vi "TrapezoidalMotionProfile.vi"(5 "MaxAccel":dbl=75.0, 7 "MaxVelocity":dbl=100.0, 8 "dt":u32=20, 9 "FinalVelocity":dbl, 10 "InitialVelocity":dbl, 11 "Distance":dbl=200.0) -> (0 "dt":u32=20, 3 "Profile":cluster{"Pos":dbl, "Vel":dbl, "Accel":dbl}[](array[cluster]))   [LabVIEW 2016]
panel:
  out "Graph":dbl[][](graph)=[[0.0, 0.015000000000000001, 0.060000000000000005, 0.135, 0.24000000000000002, 0.37500000000000006, 0.54, 0.7350000000000001, 0.9600000000000001, 1.2149999999999999, 1.5000000000000002, 1.815, 2.16, 2.535, 2.9400000000000004, 3.375, 3.8400000000000003, 4.335000000000001, 4.859999999999999, 5.415, 6.000000000000001, 6.614999999999999, 7.26, 7.9350000000000005, 8.64, 9.375, 10.14, 10.935, 11.760000000000002, 12.614999999999998, 13.5, 14.415000000000001, 15.360000000000001, 16.335, 17.340000000000003, 18.375000000000004, 19.439999999999998, 20.535, 21.66, 22.815, 24.000000000000004, 25.215000000000003, 26.459999999999997, 27.734999999999996, 29.04, 30.375000000000004, 31.740000000000002, 33.135000000000005, 34.56, 36.015, 37.5, 39.015, 40.56, 42.135000000000005, 43.74, 45.37500000000001, 47.040000000000006, 48.735000000000014, 50.459999999999994, 52.214999999999996, 54.0, 55.815, 57.660000000000004, 59.535000000000004, 61.440000000000005, 63.37500000000001, 65.34, 67.33333333333334, 69.33333333333334, 71.33333333333334, 73.33333333333334, 75.33333333333333, 77.33333333333333, 79.33333333333333, 81.33333333333333, 83.33333333333333, 85.33333333333333, 87.33333333333334, 89.33333333333334, 91.33333333333334, 93.33333333333334, 95.33333333333334, 97.33333333333334, 99.33333333333334, 101.33333333333333, 103.33333333333333, 105.33333333333333, 107.33333333333333, 109.33333333333333, 111.33333333333334, 113.33333333333334, 115.33333333333334, 117.33333333333334, 119.33333333333334, 121.33333333333334, 123.33333333333334, 125.33333333333331, 127.33333333333333, 129.33333333333331, 131.33333333333331, 133.33333333333331, 135.31833333333338, 137.27333333333337, 139.19833333333338, 141.09333333333336, 142.95833333333337, 144.79333333333338, 146.59833333333336, 148.37333333333336, 150.11833333333337, 151.83333333333337, 153.51833333333337, 155.17333333333337, 156.79833333333337, 158.39333333333337, 159.95833333333337, 161.49333333333334, 162.99833333333333, 164.47333333333336, 165.91833333333335, 167.33333333333334, 168.71833333333336, 170.07333333333335, 171.39833333333334, 172.69333333333336, 173.95833333333334, 175.19333333333336, 176.39833333333337, 177.57333333333335, 178.71833333333336, 179.83333333333334, 180.91833333333335, 181.97333333333336, 182.99833333333336, 183.99333333333337, 184.95833333333334, 185.89333333333335, 186.79833333333335, 187.67333333333335, 188.51833333333335, 189.33333333333334, 190.11833333333334, 190.87333333333333, 191.59833333333333, 192.29333333333335, 192.95833333333334, 193.59333333333333, 194.19833333333335, 194.77333333333334, 195.31833333333333, 195.83333333333334, 196.31833333333333, 196.77333333333334, 197.19833333333335, 197.59333333333333, 197.95833333333334, 198.29333333333335, 198.59833333333333, 198.87333333333333, 199.11833333333334, 199.33333333333334, 199.51833333333335, 199.67333333333335, 199.79833333333335, 199.89333333333335, 199.95833333333334, 199.99333333333334, 199.99833333333333], [0.0, 1.5, 3.0, 4.5, 6.0, 7.5, 9.0, 10.500000000000002, 12.0, 13.5, 15.0, 16.5, 18.0, 19.5, 21.000000000000004, 22.5, 24.0, 25.500000000000004, 27.0, 28.5, 30.0, 31.5, 33.0, 34.5, 36.0, 37.5, 39.0, 40.5, 42.00000000000001, 43.5, 45.0, 46.5, 48.0, 49.5, 51.00000000000001, 52.50000000000001, 54.0, 55.5, 57.0, 58.5, 60.0, 61.50000000000001, 63.0, 64.5, 66.0, 67.5, 69.0, 70.5, 72.0, 73.5, 75.0, 76.5, 78.0, 79.5, 81.0, 82.5, 84.00000000000001, 85.50000000000001, 87.0, 88.5, 90.0, 91.5, 93.0, 94.5, 96.0, 97.5, 99.0, 100.0, 100.0, 100.0, 100.0, 100.0, 100.0, 100.0, 100.0, 100.0, 100.0, 100.0, 100.0, 100.0, 100.0, 100.0, 100.0, 100.0, 100.0, 100.0, 100.0, 100.0, 100.0, 100.0, 100.0, 100.0, 100.0, 100.0, 100.0, 100.0, 100.0, 100.0, 100.0, 100.0, 100.0, 98.5, 97.0, 95.5, 94.0, 92.5, 91.0, 89.49999999999999, 87.99999999999999, 86.49999999999999, 84.99999999999999, 83.49999999999999, 81.99999999999999, 80.49999999999999, 78.99999999999999, 77.49999999999997, 76.00000000000001, 74.50000000000001, 73.00000000000001, 71.5, 70.0, 68.5, 67.0, 65.5, 64.0, 62.5, 61.0, 59.5, 57.99999999999999, 56.49999999999999, 54.99999999999999, 53.49999999999999, 51.99999999999999, 50.499999999999986, 48.999999999999986, 47.499999999999986, 45.999999999999986, 44.499999999999986, 42.999999999999986, 41.49999999999998, 39.99999999999998, 38.500000000000014, 37.000000000000014, 35.500000000000014, 34.000000000000014, 32.5, 31.0, 29.5, 28.0, 26.5, 25.0, 23.5, 22.0, 20.5, 19.0, 17.5, 15.999999999999986, 14.499999999999986, 12.999999999999986, 11.499999999999986, 9.999999999999986, 8.499999999999986, 6.999999999999986, 5.499999999999986, 3.999999999999986, 2.499999999999986, 0.9999999999999716, -0.4999999999999858]]
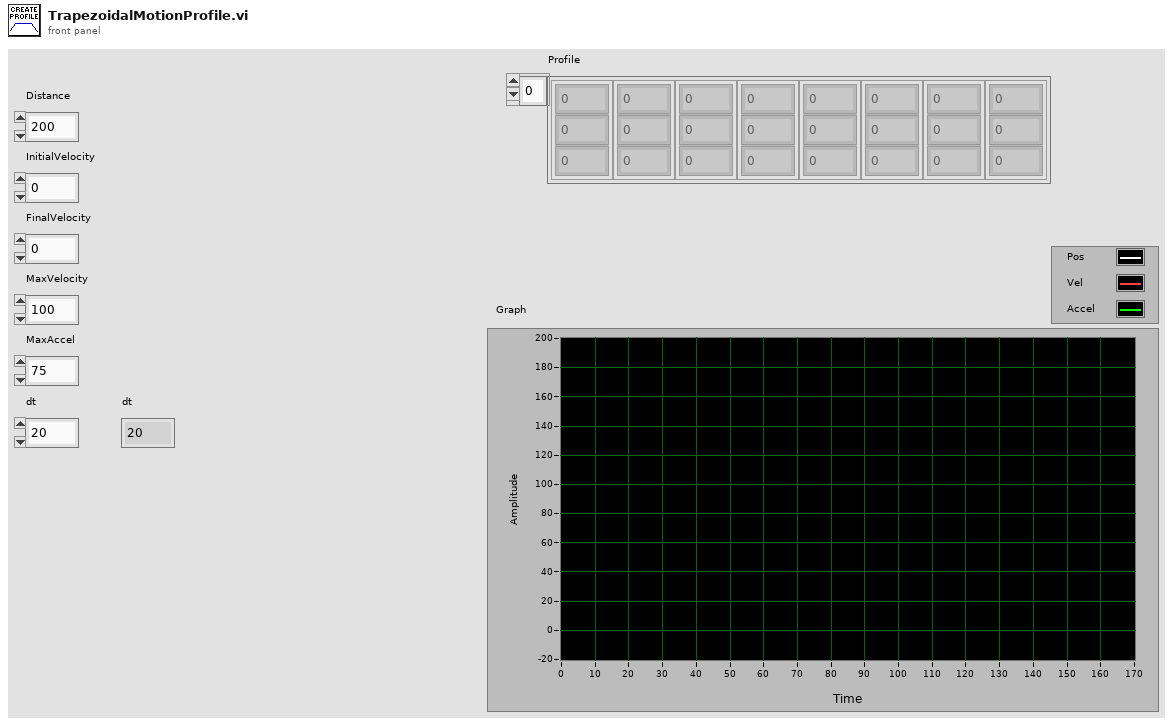
[diagram p1: front panel]
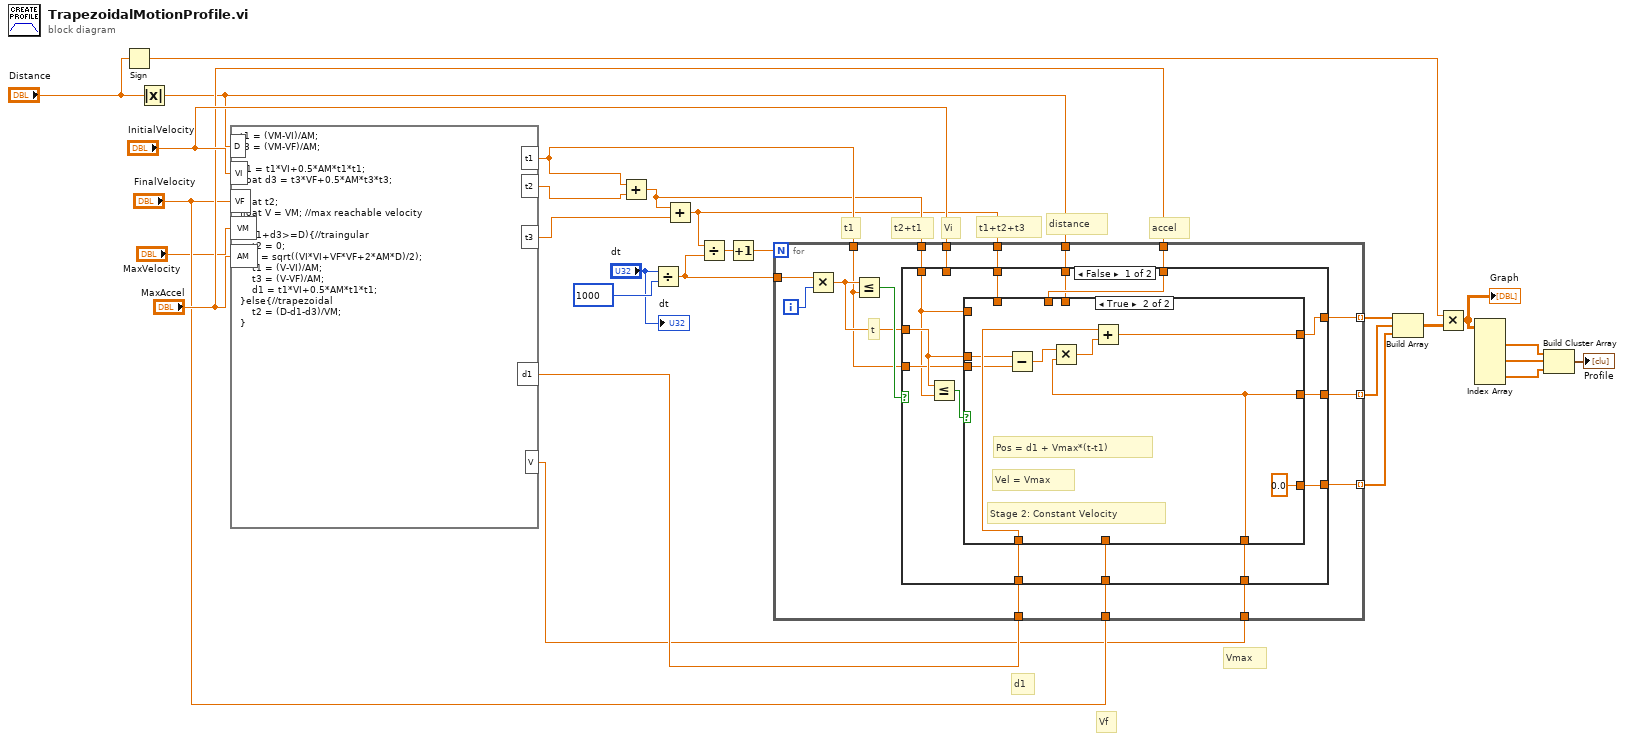
[diagram p0: block diagram]
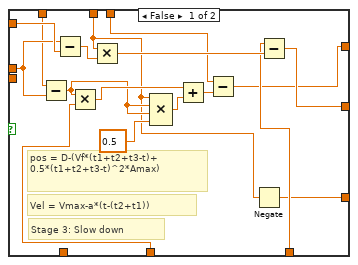
[diagram p2: hidden frame]
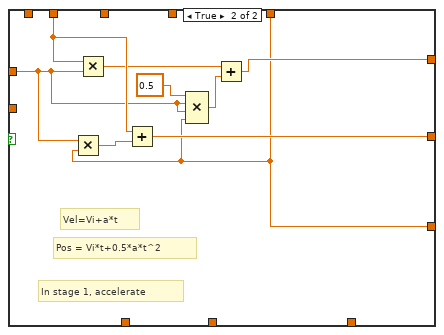
[diagram p3: hidden frame]
diagram:
  # "distance"
  # "Vf"
  # "t1+t2+t3"
  # "d1"
  # "Vmax"
  # "t1"
  # "t2+t1"
  # "Vi"
  # "accel"
  n1 = Sign(1:"Distance") -> (0:w6:dbl)
  n2 = Absolute Value(x="Distance") -> (abs(x)=w9:dbl)
  n3 = formula code="t1 = (VM-VI)/AM;\nt3 = (VM-VF)/AM;\n\nd1 = t1*VI+0.5*AM*t1*t1;\nfloat d3 = t3*VF+0.5*AM*t3*t3;\n\nfloat t2;\nfloat V = VM; //max reachable velocity\n\nif(d1+d3>=D){//traingular\n    t2 = 0;\n    V = sqrt((VI*VI+VF*VF+2*AM*D)/2);\n    t1 = (V-VI)/AM;\n    t3 = (V-VF)/AM;\n    d1 = t1*VI+0.5*AM*t1*t1;\n}else{//trapezoidal\n    t2 = (D-d1-d3)/VM;\n}"("VI"="InitialVelocity", "VF"="FinalVelocity", "D"=w9, "VM"="MaxVelocity", "AM"="MaxAccel") -> ("t1"=w22:dbl, "t3"=w27:dbl, "d1"=w18:dbl, "t2"=w28:dbl, "V"=w11:dbl)
  n4 = Add(x=w22, y=w28) -> (x+y=w19:dbl)
  n5 = Divide(x="dt", y=u32 1000) -> (x/y=w23:dbl)
  n6 = Add(x=w19, y=w27) -> (x+y=w15:dbl)
  n7 = Divide(x=w15, y=w23) -> (x/y=w25:dbl)
  n8 = Increment(x=w25) -> (x+1=w24:dbl)
  n9 = for {
    N: w24 -> [_]
    tunnel: w23 -> [w43]
    tunnel: w22 -> [w33]
    tunnel: "InitialVelocity" -> [w41]
    tunnel: "MaxAccel" -> [w40]
    tunnel: [w39] -> w16 mode=indexing
    tunnel: [w38] -> w17 mode=indexing
    tunnel: w19 -> [w37]
    tunnel: w11 -> [w35]
    tunnel: w18 -> [w34]
    tunnel: w15 -> [w32]
    tunnel: "FinalVelocity" -> [w31]
    tunnel: w9 -> [w30]
    tunnel: [w29] -> w10 mode=indexing
    i -> [w44]
    # "t"
    n10 = Multiply(x=w43, y=w44) -> (x*y=w36:dbl)
    n11 = Less Or Equal?(x=w36, y=w33) -> (x <= y?=w42:bool)
    n12 = case shown="False" w42 {
      tunnel: w41 -> [_ w89]
      tunnel: w40 -> [w49 w83]
      tunnel: w36 -> [w53 w86]
      tunnel: [w56 w90] -> w39
      tunnel: [w51 w84] -> w38
      tunnel: w37 -> [w50 _]
      tunnel: w35 -> [w55 _]
      tunnel: w34 -> [w54 _]
      tunnel: w33 -> [w52 _]
      tunnel: w32 -> [w48 _]
      tunnel: w31 -> [w47 _]
      tunnel: w30 -> [w46 _]
      tunnel: [w45 w83] -> w29
      frame False {
        n13 = Less Or Equal?(x=w53, y=w50) -> (x <= y?=w57:bool)
        n14 = case shown="True" w57 {
          tunnel: [w70 w79] -> w56
          tunnel: w55 -> [w71 w79]
          tunnel: w54 -> [_ w82]
          tunnel: w53 -> [w69 w81]
          tunnel: w52 -> [_ w80]
          tunnel: [w60 w76] -> w51
          tunnel: w50 -> [w74 _]
          tunnel: w49 -> [w58 _]
          tunnel: w48 -> [w68 _]
          tunnel: w47 -> [w67 _]
          tunnel: w46 -> [w61 _]
          tunnel: [w59 0.0] -> w45
          frame False {
            # "pos = D-(Vf*(t1+t2+t3-t)+\n0.5*(t1+t2+t3-t)^2*Amax)"
            # "Vel = Vmax-a*(t-(t2+t1))"
            # "Stage 3: Slow down"
            n15 = Subtract(x=w68, y=w69) -> (x-y=w64:dbl)
            n16 = Subtract(x=w69, y=w74) -> (x-y=w73:dbl)
            n17 = Multiply(x=w64, y=w67) -> (x*y=w66:dbl)
            n18 = Multiply(x=w58, y=w73) -> (x*y=w72:dbl)
            n19 = Compound Arithmetic op=MULTIPLY(w58, w64, w64, 0.5 ("value")) -> (w63:dbl)
            n20 = Add(x=w66, y=w63) -> (x+y=w62:dbl)
            n21 = Subtract(x=w61, y=w62) -> (x-y=w60:dbl)
            n22 = Negate(x=w58) -> (-x=w59:dbl)
            n23 = Subtract(x=w71, y=w72) -> (x-y=w70:dbl)
          }
          frame True {
            # "Pos = d1 + Vmax*(t-t1)"
            # "Vel = Vmax"
            # "Stage 2: Constant Velocity"
            n24 = Subtract(x=w81, y=w80) -> (x-y=w78:dbl)
            n25 = Multiply(x=w78, y=w79) -> (x*y=w77:dbl)
            n26 = Add(x=w82, y=w77) -> (x+y=w76:dbl)
          }
        }
      }
      frame True {
        # "Vel=Vi+a*t"
        # "Pos = Vi*t+0.5*a*t^2"
        # "In stage 1, accelerate"
        n27 = Multiply(x=w86, y=w83) -> (x*y=w91:dbl)
        n28 = Multiply(x=w89, y=w86) -> (x*y=w88:dbl)
        n29 = Add(x=w89, y=w91) -> (x+y=w90:dbl)
        n30 = Compound Arithmetic op=MULTIPLY(0.5 ("t2"), w86, w86, w83) -> (w85:dbl)
        n31 = Add(x=w88, y=w85) -> (x+y=w84:dbl)
      }
    }
  }
  n32 = Build Array(w17, w16, w10) -> (w7:dbl[][])
  n33 = Multiply(x=w6, y=w7) -> (x*y=w5:dbl[][])
  "Graph" <- w5
  n34 = Index Array(array=w5) -> (element #1=w4:dbl[], element #2=w3:dbl[], element #3=w2:dbl[])  [unwired: 6 in]
  n35 = Build Cluster Array(w4, w3, w2) -> (→"Profile":cluster{dbl, dbl, dbl}[])
  "dt" <- "dt"
